vi "VI Server_Signaling_Set Text Ring by Item Selected.vi"(7 "Label":string, 8 "error in":errorcluster, 9 "Item":string, 11 "VI Server Cluster":T1={"Labels"=["Label", "Size", "Font", "Heght", "Width", "Ledding Denominator", "Ledding Nominator", "Label Number", "Microstep Resolution", "X", "Y", "Z", "Italic?", "Underlined?"], "Refs"=[], "VI Ref"=refnum}) -> (0 "error out":errorcluster, 1 "Control Reference":refnum<vi>, 3 "VI Server Cluster.DUP":T1={"Labels"=["Label", "Size", "Font", "Heght", "Width", "Ledding Denominator", "Ledding Nominator", "Label Number", "Microstep Resolution", "X", "Y", "Z", "Italic?", "Underlined?"], "Refs"=[], "VI Ref"=refnum})   [LabVIEW 2020]
doc: "Sets value of Text Ring control/indicator by Item name and places it into user events queue."
uses:
  VI Server_TypeDefs/VI Server_RefsCluster.ctl
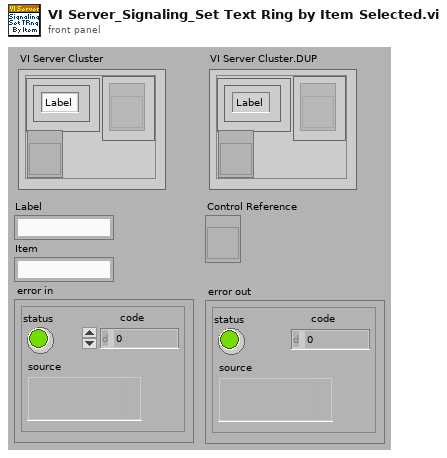
[diagram p1: front panel]
types:
  T1 = typedef "VI Server_RefsCluster.ctl" = cluster{"Labels":string[], "Refs":refnum<vi>[], "VI Ref":refnum<vi>}
  T2 = typedef "LVStringsAndValuesArrayTypeDef_U16.ctl" = cluster{"String":string, "Value":u16}[]
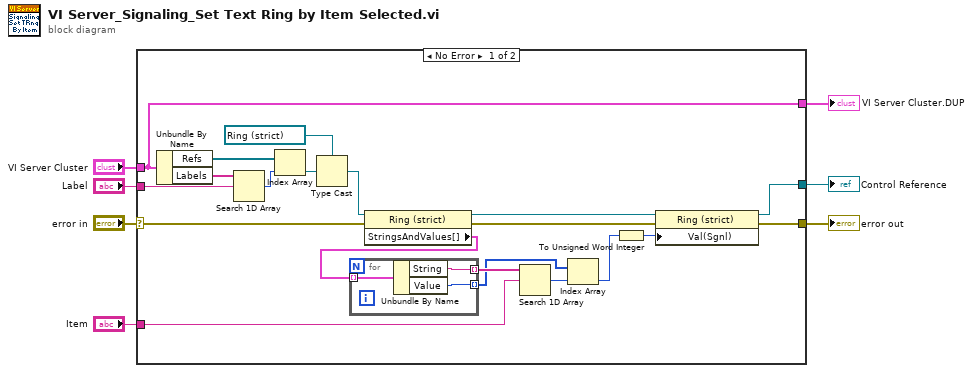
[diagram p0: block diagram]
diagram:
  n1 = case shown="No Error" "error in" {
    selector: "error in" -> [w21 w31]
    tunnel: "Label" -> [w26 _]
    tunnel: "VI Server Cluster" -> [w8 _]
    tunnel: [w18 w31] -> w7
    tunnel: [w15 _] -> w3
    tunnel: "Item" -> [w20 _]
    tunnel: [w8 _] -> w1
    frame No Error {
      n2 = Unbundle By Name(w8) -> ("Refs"=w24:refnum<vi>[], "Labels"=w27:string[])
      n3 = Search 1D Array(1D array=w27, element=w26) -> (index of element=w25:i32)  [unwired: 1 out]
      n4 = Index Array(array=w24, index=w25) -> (element=w23:refnum<vi>)
      n5 = Type Cast(type=refnum<vi> refnum ("Ring"), x=w23) -> (*(type *) &x=w16:refnum<vi>)
      n6 = property class="Ring (strict)"(reference=w16, error in=w21) -> (reference out=w17:refnum<vi>, error out=w19:errorcluster, "StringsAndValues[]"=w13:T2)
      n7 = for {
        tunnel: w13 -> [w30] mode=indexing
        tunnel: [w29] -> w12 mode=indexing
        tunnel: [w28] -> w11 mode=indexing
        n8 = Unbundle By Name(w30) -> ("String"=w29:string, "Value"=w28:u16)
      }
      n9 = Search 1D Array(1D array=w12, element=w20) -> (index of element=w10:i32)  [unwired: 1 out]
      n10 = Index Array(array=w11, index=w10) -> (element=w9:u16)
      n11 = To Unsigned Word Integer(number=w9) -> (unsigned 16bit integer=w14:u16)
      n12 = property class="Ring (strict)"(reference=w17, error in=w19, "Val(Sgnl)"=w14) -> (reference out=w15:refnum<vi>, error out=w18:errorcluster)
    }
    frame Error {
    }
  }
  "error out" <- w7
  "VI Server Cluster.DUP" <- w1
  "Control Reference" <- w3
